vi "Einheiten finden.vi"(10 "Komponente":u16, 11 "Aktuelle Gasliste gesamt":T1[](array[typedef])) -> (0 "Einheit in String":string, 1 "Komponenten Name":T1)   [LabVIEW 2020, in "Gaszuordnung AO.lvlib"]
uses:
  Gaszuordnung AO.lvlib
  Visualisierungs Elemente/String - Ausgabefeld.ctl
  FGV Gaszuordnung Grenzen&Einheit Aktion.ctl
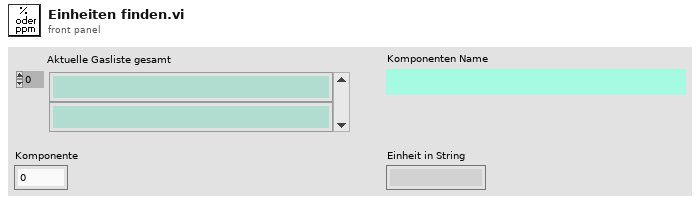
[diagram p1: front panel]
types:
  T1 = typedef "String - Ausgabefeld.ctl" = string
  T2 = typedef "Gaszuordnung AO.lvlib/FGV Gaszuordnung Grenzen&Einheit Aktion.ctl" = enum16{"Lesen", "Schreiben Min", "Schreiben Max", "Laden", "Speichern"}
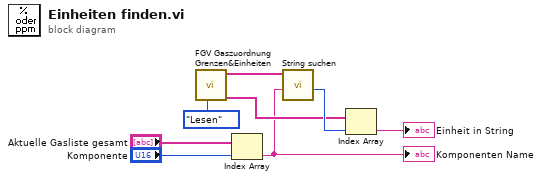
[diagram p0: block diagram]
diagram:
  n1 = call "FGV Gaszuordnung Grenzen&Einheiten.vi"("Aktion"=FGV_Gaszuordnung_Grenzen&Einheit_Aktion."Lesen") -> ("Einheit neu"=w6:string[], "Namen neu"=w3:string[])  [unwired: 7 in, 2 out]
  n2 = Index Array(array="Aktuelle Gasliste gesamt", index="Komponente") -> (element=w2:T1)
  "Komponenten Name" <- w2
  n3 = call "String suchen.vi"("Gasname"=w2, "Such-Namen"=w3) -> ("Index"=w7:i32)  [unwired: 8 in, 1 out]
  n4 = Index Array(array=w6, index=w7) -> (element=→"Einheit in String":string)
